vi "Open_connection.vi"(8 "error in (no error)":errorcluster, 11 "DB_SQLite in":refnum<class "DB_SQLite.lvclass">) -> (0 "error out":errorcluster, 3 "DB_SQLite out":refnum<class "DB_SQLite.lvclass">)   [LabVIEW 2015, in "DB_SQLite.lvclass"]
uses:
  DB_SQLite.lvclass
  DB.lvclass/DB.ctl
  <vilib>/drjdpowell/SQLite Library/SQL Connection/Open (path).vi
  <vilib>/drjdpowell/SQLite Library/SQL Connection/Open (string).vi
  <vilib>/AdvancedString/Path To Command Line String.vi
  <vilib>/drjdpowell/SQLite Library/SQL Connection/Connection.lvclass
  DB.lvclass
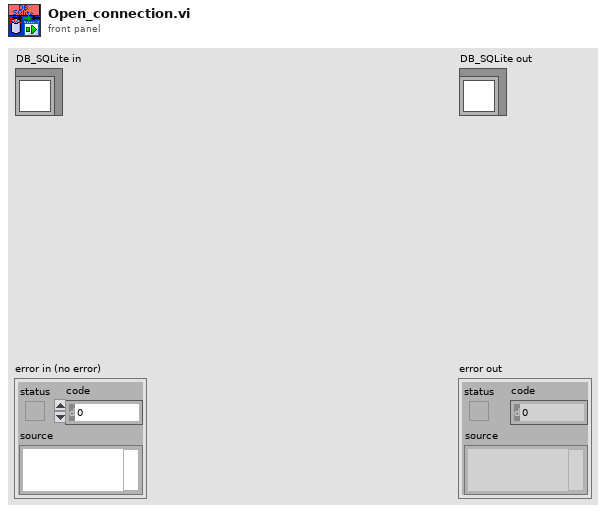
[diagram p1: front panel]
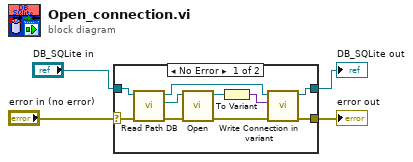
[diagram p0: block diagram]
diagram:
  n1 = case shown="No Error" "error in (no error)" {
    selector: "error in (no error)" -> [w11 w16]
    tunnel: [w5 w16] -> w3
    tunnel: [w8 w15] -> w2
    tunnel: "DB_SQLite in" -> [w12 w15]
    frame No Error {
      n2 = call "Read Path DB.vi"("error in (no error)"=w11, "DB in"=w12) -> ("error out"=w13:errorcluster, "Path DB"=w14:path, "DB out"=w9:refnum<class "DB_SQLite.lvclass">)  [unwired: 7 in]
      n3 = call-poly <vilib>:"Open.vi"("error in (no error)"=w13, "db file"=w14) -> ("error out"=w6:errorcluster, "SQLite Connection"=w10:refnum<class "Connection.lvclass">)  [unwired: 8 in]
      n4 = To Variant(anything=w10) -> (Variant=w7:variant)
      n5 = call "Write Connection in variant.vi"("error in (no error)"=w6, "Connection in variant"=w7, "DB in"=w9) -> ("error out"=w5:errorcluster, "DB out"=w8:refnum<class "DB_SQLite.lvclass">)  [unwired: 7 in]
    }
    frame Error {
    }
  }
  "error out" <- w3
  "DB_SQLite out" <- w2
